vi "Destroy A Rendezvous.vi"(4 "error in (no error)":errorcluster, 7 "rendezvous":T1) -> (0 "error out":errorcluster, 3 "rendezvous name":string)   [LabVIEW 2010]
doc: "Destroys the specified rendezvous."
uses:
  RendezvousDataCluster.ctl
panel:
  in  "Error Message":string="Attempted to release an invalid rendezvous reference."
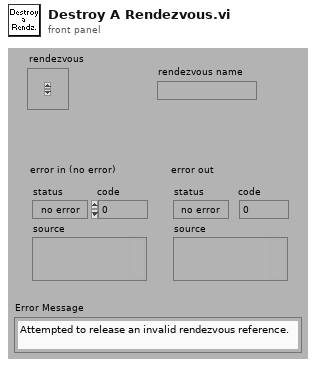
[diagram p1: front panel]
types:
  T1 = typedef "Rendezvous RefNum" = refnum<k1>
  T2 = typedef "RendezvousDataCluster.ctl" = cluster{"Threshold":i32, "Messenger Queues":refnum<queue>[]}
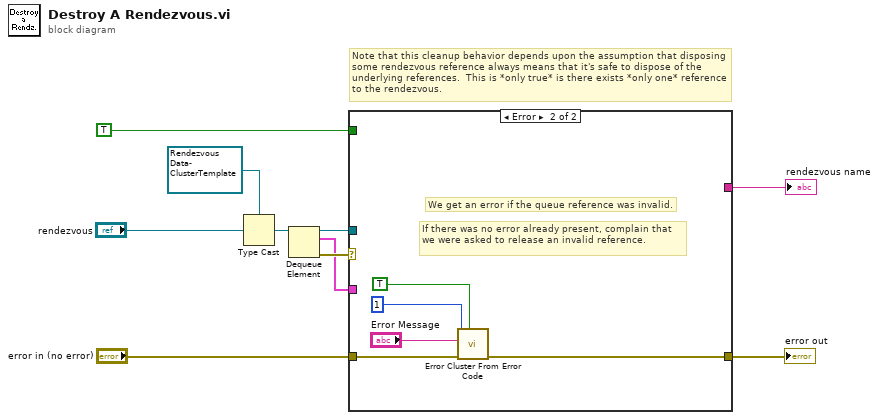
[diagram p0: block diagram]
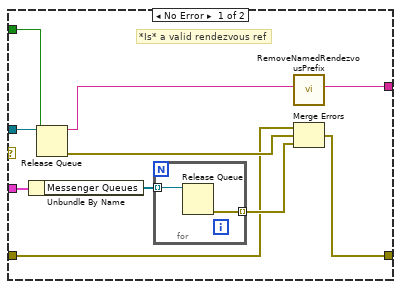
[diagram p2: hidden frame]
diagram:
  # "Note that this cleanup behavior depends upon the assumption that disposing some rendezvous reference always means that it's safe to dispose of the underlying references.  This is *only true* is there exists *only one* reference to the rendezvous."
  n1 = Type Cast(type=refnum<queue> refnum ("queue out"), x="rendezvous") -> (*(type *) &x=w9:refnum<queue>)
  n2 = Dequeue Element(queue=w9) -> (queue out=w7:refnum<queue>, element=w6:T2, error out=w8:errorcluster)  [unwired: 1 in, 2 out]
  n3 = case shown="Error" w8 {
    tunnel: [w13 w27] -> w2
    tunnel: w7 -> [w17 _]
    tunnel: w6 -> [w16 _]
    tunnel: "error in (no error)" -> [w15 w23]
    tunnel: TRUE -> [w14 _]
    tunnel: [w12 _] -> w3
    frame No Error {
      # "*Is* a valid rendezvous ref"
      n4 = Unbundle By Name(w16) -> ("Messenger Queues"=w18:refnum<queue>[])
      n5 = Release Queue(queue=w17, force destroy? (F)=w14) -> (queue name=w11:string, error out=w20:errorcluster)  [unwired: 1 in, 1 out]
      n6 = for {
        tunnel: w18 -> [w22] mode=indexing
        tunnel: [w21] -> w19 mode=indexing
        n7 = Release Queue(queue=w22) -> (error out=w21:errorcluster)  [unwired: 1 in, 3 out]
      }
      n8 = call "RemoveNamedRendezvousPrefix.vi"("Name In"=w11) -> ("Name Out"=w12:string)  [unwired: 10 out]
      n9 = Merge Errors(w15, w20, w19) -> (w13:errorcluster)
    }
    frame Error {
      # "We get an error if the queue reference was invalid."
      # "If there was no error already present, complain that we were asked to release an invalid reference."
      n10 = call "Error Cluster From Error Code.vi"("show call chain? (False)"=TRUE, "error in (no error)"=w23, "error message (\"\")"="Error Message", "error code (0)"=1) -> ("error out"=w27:errorcluster)  [unwired: 5 out]
    }
  }
  "rendezvous name" <- w3
  "error out" <- w2
